vi "AIM664 Command TX Port Init.vi"() -> ()   [LabVIEW 2020]
uses:
  AIM664LV.lvlib
panel:
  out "error out":errorcluster
  out "BSP Version Out":T1
  out "BSP Version Out":T1
  in  "FdxLogin":T2={"SrvName"="local", "ClHostName"="local", "ClUser"="Brett", "ClApplication"="Test", "ClApplicationVersion"="V01.00", "ResourceID"=1, "Privileges"=4294967295} {"Privileges" min=4294967295 format="%x"}
  out "NuOfServers":u32
  # "ARINC 664 Initialize Tx Port"
  # "Overview: Initialize Tx Port of the boards available in a system and present some properties of those resources.\nRequirement: At least one AIM ARINC-664 board with installed AIM ARINC 664 BSP.\nRestrictions: None.\nInstruction:\n1. Run the VI.\n2. Verify the resources available. If no error is presented, you will see all of the resources in the Resources."
  # "FdxInit Test"
  # "FdxLogin"
  # "FdxReadBSPVersion"
  # "FdxLogout"
  # "FdxReadBSPVersionSpecial"
  # "Output"
  # "Input"
  # "Output"
  # "Output"
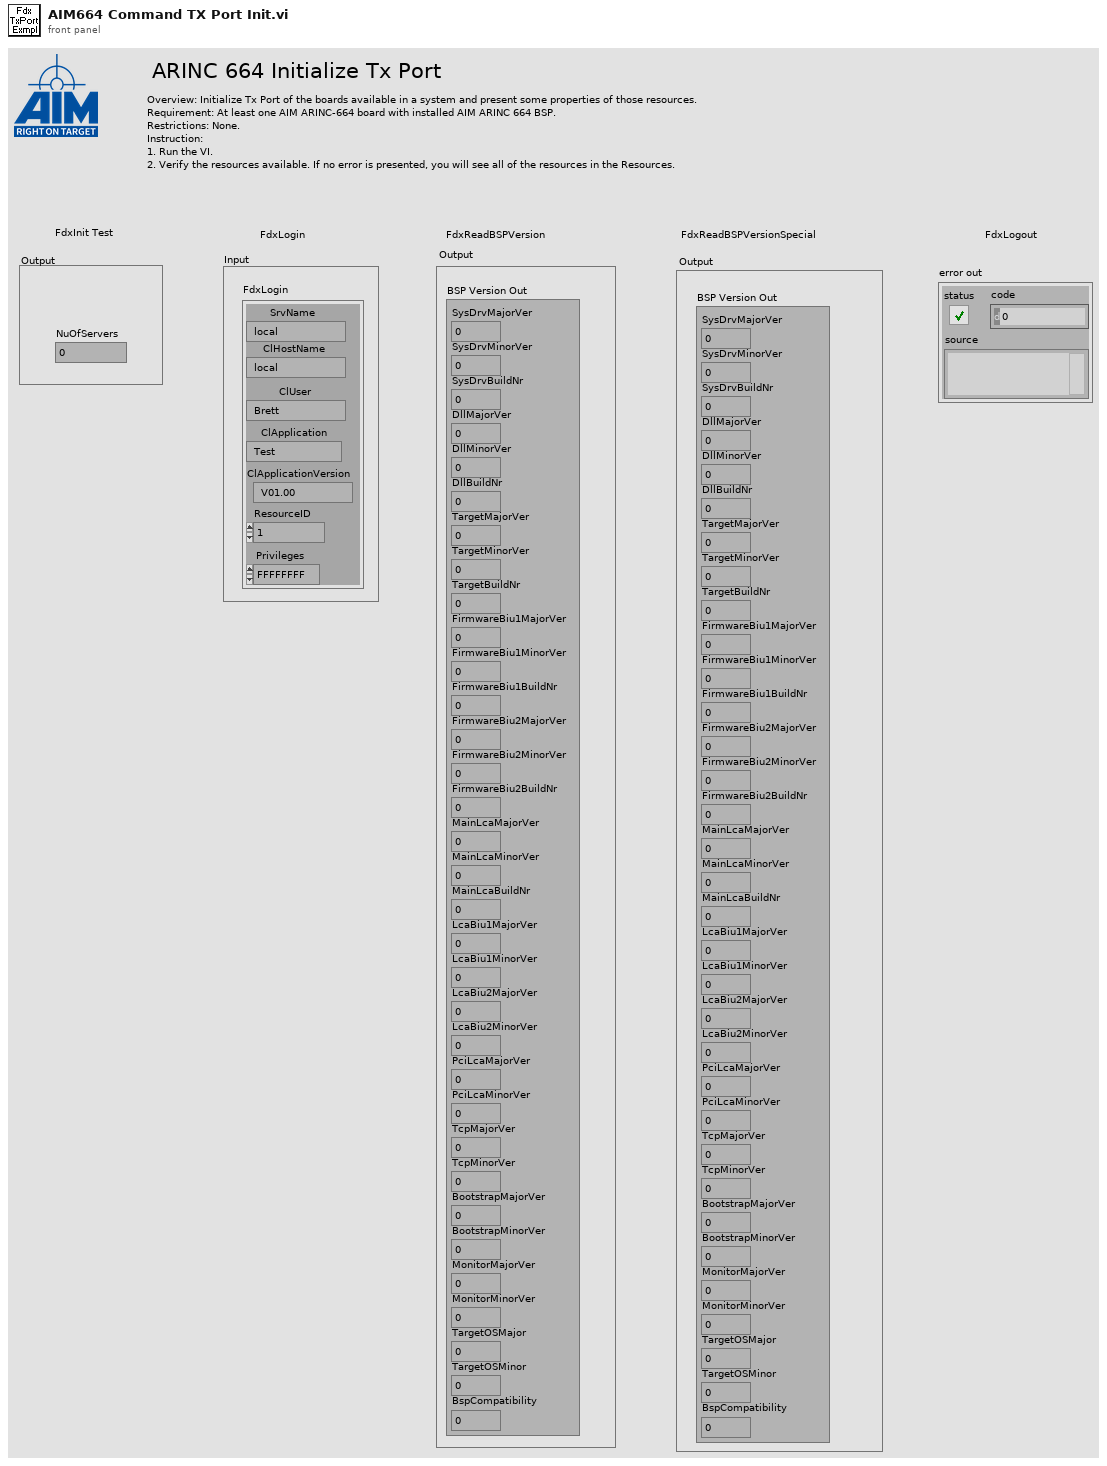
[diagram p1: front panel]
types:
  T1 = cluster{"SysDrvMajorVer":u32, "SysDrvMinorVer":u32, "SysDrvBuildNr":u32, "DllMajorVer":u32, "DllMinorVer":u32, "DllBuildNr":u32, "TargetMajorVer":u32, "TargetMinorVer":u32, "TargetBuildNr":u32, "FirmwareBiu1MajorVer":u32, "FirmwareBiu1MinorVer":u32, "FirmwareBiu1BuildNr":u32, "FirmwareBiu2MajorVer":u32, "FirmwareBiu2MinorVer":u32, "FirmwareBiu2BuildNr":u32, "MainLcaMajorVer":u32, "MainLcaMinorVer":u32, "MainLcaBuildNr":u32, "LcaBiu1MajorVer":u32, "LcaBiu1MinorVer":u32, "LcaBiu2MajorVer":u32, "LcaBiu2MinorVer":u32, "PciLcaMajorVer":u32, "PciLcaMinorVer":u32, "TcpMajorVer":u32, "TcpMinorVer":u32, "BootstrapMajorVer":u32, "BootstrapMinorVer":u32, "MonitorMajorVer":u32, "MonitorMinorVer":u32, "TargetOSMajor":u32, "TargetOSMinor":u32, "BspCompatibility":u32}
  T2 = cluster{"SrvName":string, "ClHostName":string, "ClUser":string, "ClApplication":string, "ClApplicationVersion":string, "ResourceID":u32, "Privileges":u32}
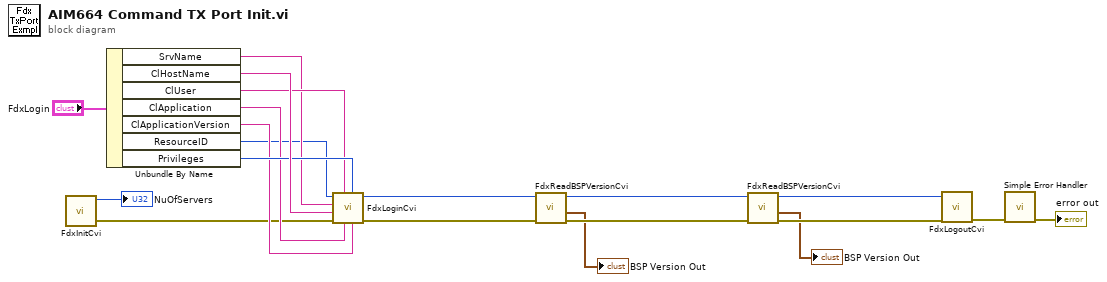
[diagram p0: block diagram]
diagram:
  n1 = call "FdxInitCvi.vi"() -> ("error out"=w7:errorcluster, "Number of Servers"=→"NuOfServers":u32)  [unwired: 10 in]
  n2 = Unbundle By Name("FdxLogin") -> ("SrvName"=w10:string, "ClHostName"=w15:string, "ClUser"=w13:string, "ClApplication"=w12:string, "ClApplicationVersion"=w11:string, "ResourceID"=w9:u32, "Privileges"=w14:u32)
  n3 = call "FdxLoginCvi.vi"("ClApplicationVersion"=w11, "Privileges"=w14, "ClApplication"=w12, "ClUser"=w13, "error in"=w7, "ClHostName"=w15, "SrvName"=w10, "ResourceID"=w9) -> ("error out"=w8:errorcluster, "InstrumentHandle"=w5:u32)  [unwired: 2 in]
  n4 = call "FdxReadBSPVersionCvi.vi"("error in"=w8, "InstrumentHandle_board in"=w5) -> ("error out"=w20:errorcluster, "BSP Version Out"=→"BSP Version Out":T1, "InstrumentHandle_board out"=w4:u32)  [unwired: 7 in]
  n5 = call "FdxReadBSPVersionCvi.vi"("error in"=w20, "InstrumentHandle_board in"=w4) -> ("error out"=w19:errorcluster, "BSP Version Out"=→"BSP Version Out":T1, "InstrumentHandle_board out"=w3:u32)  [unwired: 7 in]
  n6 = call "FdxLogoutCvi.vi"("error in"=w19, "InstrumentHandle"=w3) -> ("error out"=w2:errorcluster)  [unwired: 9 in]
  n7 = call <vilib>:"Simple Error Handler.vi"("error in (no error)"=w2) -> ("error out"=→"error out":errorcluster)  [unwired: 4 in, 4 out]
